vi "Log View for Power Spectrum.vi"(2 "channel info":T1={"sensor sensitivity [mV/EU]"=1000.0, "engineering units"=1, "dB reference [EU]"=1.0, "custom label"="EU", "weighting filter"=0, "pregain [dB]"=0.0} {"pregain [dB]" format="%.2f"; "weighting filter" items=["Linear", "A-weighting", "B-weighting", "C-weighting", "ITU-R 468-4", "Dolby", "CCITT", "C-message"]; "dB reference [EU]" format="%^.1e"; "engineering units" items=["custom..."=0, "V"=1, "A"=21, "Pa"=2, "N"=20, "g"=3, "m/s^2"=4, "m/s"=5, "m"=6, "mm/s"=12, "mm"=13, "microns/s"=14, "microns"=15, "in/s^2"=7, "in/s"=8, "in"=9, "mils/s"=10, "mils"=11, "rad/s^2"=16, "rad/s"=17, "rad"=18, "strain"=19]; "sensor sensitivity [mV/EU]" format="%.2f"}, 4 "dB On (T)":bool=TRUE, 5 "power spectrum [EU^2 rms]":dbl[](array[numeric]) format="%.2f") -> (0 "unit label":string, 1 "log view power spectrum [dB EU]":dbl[](array[numeric]) format="%.2f")   [LabVIEW 2017]
uses:
  <vilib>/addons/Sound and Vibration/compatibility/Controls/svl_Channel Info.ctl
  <vilib>/addons/Sound and Vibration/compatibility/Controls/svl_Engineering Units Text Ring.ctl
  <vilib>/addons/Sound and Vibration/compatibility/Controls/svl_Weighting Filter Text Ring.ctl
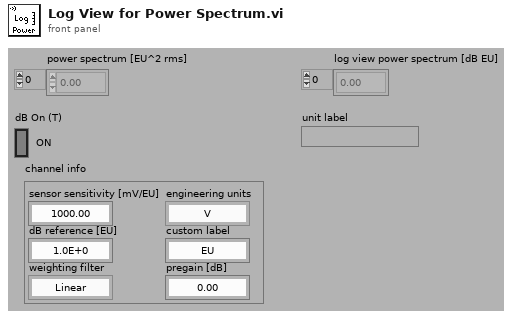
[diagram p1: front panel]
types:
  T1 = typedef "svl_Channel Info.ctl" = cluster{"sensor sensitivity [mV/EU]":dbl, "engineering units":T2, "dB reference [EU]":dbl, "custom label":string, "weighting filter":T3, "pregain [dB]":dbl}
  T2 = typedef "svl_Engineering Units Text Ring.ctl" = u16
  T3 = typedef "svl_Weighting Filter Text Ring.ctl" = u16
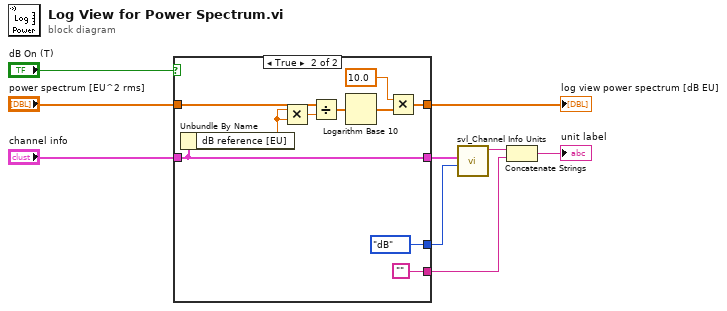
[diagram p0: block diagram]
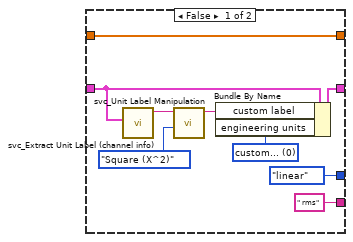
[diagram p2: hidden frame]
diagram:
  n1 = case shown="True" "dB On (T)" {
    tunnel: [w18 w25] -> w6
    tunnel: "power spectrum [EU^2 rms]" -> [w18 w27]
    tunnel: "channel info" -> [w14 w24]
    tunnel: [w13 w24] -> w3
    tunnel: [" rms" ""] -> w2
    tunnel: [enum16{"linear", "dB"}."linear" ("linear/dB") enum16{"linear", "dB"}."dB" ("linear/dB")] -> w1
    frame False {
      w11 = u16 0 items=["custom...", "V", "Pa", "g", "m/s^2", "m/s", "m", "in/s^2", "in/s", "in", "mm", "mils", "A"] ("engineering units")
      n2 = call <vilib>:"svc_Extract Unit Label (channel info).vi"("channel info"=w14) -> ("unit label"=w16:string)  [unwired: 8 in, 2 out]
      n3 = call <vilib>:"svc_Unit Label Manipulation.vi"("operation"=enum16{"Square (X^2)", "Divide (X/Y)"}."Square (X^2)", "X unit label"=w16) -> ("resulting unit label"=w12:string)  [unwired: 5 in]
      n4 = Bundle By Name(cluster=w14, "custom label"=w12, "engineering units"=w11) -> (w13:T1)
    }
    frame True {
      n5 = Unbundle By Name(w24) -> ("dB reference [EU]"=w23:dbl)
      n6 = Multiply(x=w23, y=w23) -> (x*y=w26:dbl)
      n7 = Divide(x=w27, y=w26) -> (x/y=w28:dbl[])
      n8 = Logarithm Base 10(1:w28) -> (0:w21:dbl[])
      n9 = Multiply(x=10.0 ("y"), y=w21) -> (x*y=w25:dbl[])
    }
  }
  "log view power spectrum [dB EU]" <- w6
  n10 = call <vilib>:"svl_Channel Info Units.vi"("linear/dB"=w1, "channel info"=w3) -> ("unit label"=w5:string)  [unwired: 8 in, 1 out]
  n11 = Concatenate Strings(w5, w2) -> (→"unit label":string)
